vi "Initialize Notifier.vi"(8 "error in":errorcluster) -> (0 "error out":errorcluster)   [LabVIEW 2020, in "Sequencer Handshake.lvlib"]
uses:
  Sequencer Handshake.lvlib
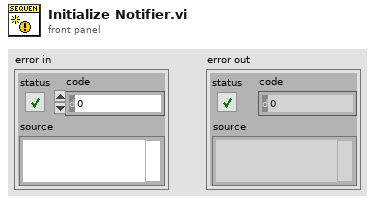
[diagram p1: front panel]
types:
  T1 = enum16{"Obtain", "Send", "Get Notifier", "Release"}
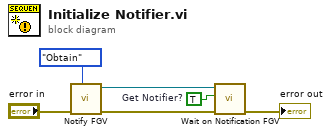
[diagram p0: block diagram]
diagram:
  w3 = TRUE  # Get Notifier?
  n1 = call "Notify FGV.vi"("Actions"=T1."Obtain", "error in"="error in") -> ("error out"=w4:errorcluster, "notifier out"=w5:refnum<notifier>)  [unwired: 8 in]
  n2 = call "Wait on Notification FGV.vi"("error in"=w4, "Get Notifier?"=w3, "notifier in"=w5) -> ("error out"=→"error out":errorcluster)  [unwired: 6 in, 2 out]
